vi "StateHapticEngine.vi"(0 "Master State":enum16{"Normal", "Climb"}(ring)) -> ()   [LabVIEW 2020]
doc: "Manages the haptic feedback on the driver and manipulator joysticks."
uses:
  refnumbers.vi
  GRNF_Joystick.vi
  driverdata.vi
  autonomousinfo.vi
  robotoutputs.vi
  drivercommands.vi
  sensordata.vi
panel:
  in  "Develop New Haptic":bool
  in  "Duty Cycle (%)":dbl=100.0
  in  "Amplitude":dbl=1.0
  in  "Period (s)":dbl=10.0
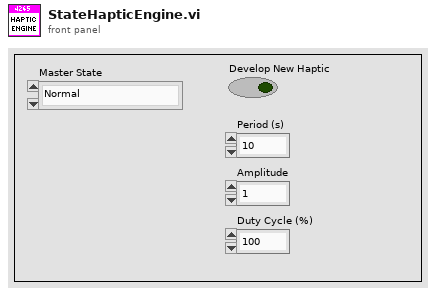
[diagram p1: front panel]
types:
  T1 = enum16{"None", "Development", "Longpress Buttons", "Intake", "Firing"}
  T2 = typedef "WPI_JoystickDevRef.ctl" = cluster{"Device":T3}
  T3 = typedef "WPI_JoystickDeviceEnum.ctl" = enum16{"USB 0", "USB 1", "USB 2", "USB 3", "USB 4", "USB 5"}
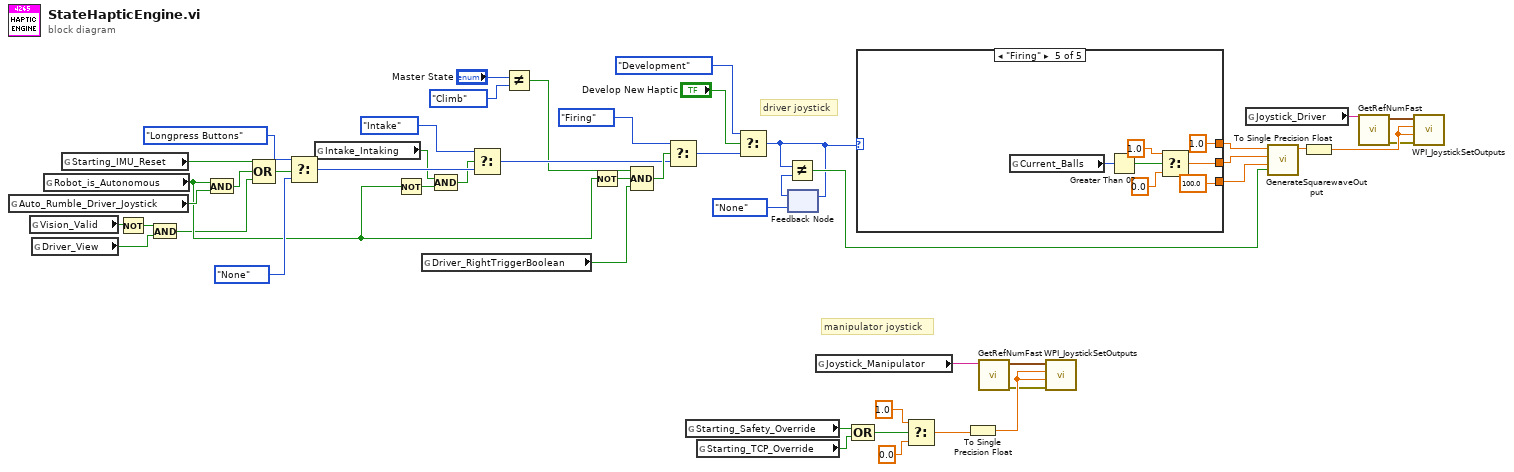
[diagram p0: block diagram]
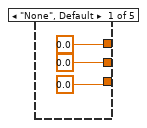
[diagram p2: hidden frame]
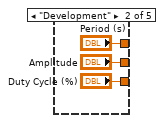
[diagram p3: hidden frame]
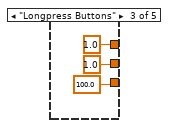
[diagram p4: hidden frame]
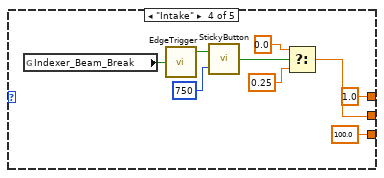
[diagram p5: hidden frame]
diagram:
  # "manipulator joystick"
  # "driver joystick"
  n1 = global read "autonomousinfo.vi" "Auto_Rumble_Driver_Joystick"() -> (w35:bool)
  n2 = global read "sensordata.vi" "Vision_Valid"() -> (w9:bool)
  n3 = global read "drivercommands.vi" "Driver_View"() -> (w7:bool)
  n4 = global read "driverdata.vi" "Robot_is_Autonomous"() -> (w11:bool)
  n5 = global read "driverdata.vi" "Starting_IMU_Reset"() -> (w37:bool)
  n6 = Not(x=w9) -> (.not. x?=w8:bool)
  n7 = And(x=w8, y=w7) -> (x .and. y?=w6:bool)
  n8 = And(x=w11, y=w35) -> (x .and. y?=w34:bool)
  n9 = Compound Arithmetic op=OR(w37, w34, w6) -> (w32:bool)
  n10 = Select(t=T1."Longpress Buttons", s=w32, f=T1."None") -> (s? t:f=w23:T1)
  n11 = global read "robotoutputs.vi" "Intake_Intaking"() -> (w18:bool)
  n12 = Not(x=w11) -> (.not. x?=w17:bool)
  n13 = global read "drivercommands.vi" "Driver_RightTriggerBoolean"() -> (w5:bool)
  n14 = Compound Arithmetic op=AND(w18, w17) -> (w16:bool)
  n15 = Select(t=T1."Intake", s=w16, f=w23) -> (s? t:f=w12:T1)
  n16 = Not Equal?(x="Master State", y=enum16{"Normal", "Climb"}."Climb") -> (x != y?=w2:bool)
  n17 = Not(x=w11) -> (.not. x?=w14:bool)
  n18 = Compound Arithmetic op=AND(w2, w14, w5) -> (w13:bool)
  n19 = Select(t=T1."Firing", s=w13, f=w12) -> (s? t:f=w10:T1)
  n20 = global read "driverdata.vi" "Starting_Safety_Override"() -> (w36:bool)
  n21 = global read "driverdata.vi" "Starting_TCP_Override"() -> (w1:bool)
  n22 = Select(t=T1."Development", s="Develop New Haptic", f=w10) -> (s? t:f=w24:T1)
  n23 = feedback-in #1(w24) -> ()
  n24 = feedback #1(T1."None") -> (w27:T1)
  n25 = Not Equal?(x=w24, y=w27) -> (x != y?=w26:bool)
  n26 = global read "refnumbers.vi" "Joystick_Manipulator"() -> (w38:string)
  n27 = Compound Arithmetic op=OR(w36, w1) -> (w44:bool)
  n28 = case shown="\"Firing\"" w24 {
    tunnel: [0.0 ("Period (s)") "Period (s)" 1.0 ("Period (s)") 1.0 ("Period (s)") 1.0 ("Period (s)")] -> w21
    tunnel: [0.0 ("Amplitude") "Amplitude" 1.0 ("Amplitude") w61 w70] -> w20
    tunnel: [0.0 ("Duty Cycle (%)") "Duty Cycle (%)" 100.0 ("Duty Cycle (%)") 100.0 ("Duty Cycle (%)") 100.0 ("Duty Cycle (%)")] -> w19
    frame "None", Default {
    }
    frame "Development" {
    }
    frame "Longpress Buttons" {
    }
    frame "Intake" {
      n29 = global read "sensordata.vi" "Indexer_Beam_Break"() -> (w67:bool)
      n30 = call "EdgeTrigger.vi"("Input Signal"=w67) -> ("Rising Edge Trigger"=w65:bool)  [unwired: 2 out]
      n31 = call "StickyButton.vi"("Time threshold (ms)"=u32 750, "Button Input"=w65) -> ("Sticky Button"=w63:bool)
      n32 = Select(t=0.0, s=w63, f=0.25) -> (s? t:f=w61:dbl)
    }
    frame "Firing" {
      n33 = global read "sensordata.vi" "Current_Balls"() -> (w69:i16)
      n34 = Greater Than 0?(x=w69) -> (x > 0?=w68:bool)
      n35 = Select(t=1.0, s=w68, f=0.0) -> (s? t:f=w70:dbl)
    }
  }
  n36 = Select(t=1.0, s=w44, f=0.0) -> (s? t:f=w46:dbl)
  n37 = To Single Precision Float(number=w46) -> (single precision float=w45:sgl)
  n38 = call-poly "GetRefNumFast.vi"("RefNum Name"=w38) -> ("Error"=w40:errorcluster, "Device Reference"=w39:T2)  [unwired: 5 in]
  n39 = call <vilib>:"WPI_JoystickSetOutputs.vi"("error in (no error)"=w40, "Right Rumble"=w45, "Left Rumble"=w45, "JoystickDevRef"=w39) -> ()  [unwired: 6 in, 2 out]
  n40 = global read "refnumbers.vi" "Joystick_Driver"() -> (w41:string)
  n41 = call "GenerateSquarewaveOutput.vi"("Init"=w26, "Duty Cycle (%)"=w19, "Amplitude"=w20, "Period (s)"=w21) -> ("Square Wave Ouput"=w33:dbl)  [unwired: 7 in]
  n42 = To Single Precision Float(number=w33) -> (single precision float=w49:sgl)
  n43 = call-poly "GetRefNumFast.vi"("RefNum Name"=w41) -> ("Error"=w42:errorcluster, "Device Reference"=w43:T2)  [unwired: 5 in]
  n44 = call <vilib>:"WPI_JoystickSetOutputs.vi"("error in (no error)"=w42, "Right Rumble"=w49, "Left Rumble"=w49, "JoystickDevRef"=w43) -> ()  [unwired: 6 in, 2 out]
